vi "RoundU8.vi"(5 "Decimal places":i8, 6 "Number":u8) -> (2 "Rounded number":u8)   [LabVIEW 2017, in "GPNumeric.lvlib"]
doc: "Rounds <B>Number</B> to a number of <B>Decimal places</B>.\n\nSet <B>Decimal places</B> to a negative number to round to nearest 10, nearest 100 and so on. E.g. to round 782 to the nearest hundred, you set <B>Decimal places</B> to -2 and the <B>Rounded number</B> will be 800.\n\nThis VI is inlined.\n\n<B>Note</B> This VI uses the default IEEE 754 round-half-to-even rounding mode.\n\nSteen Schmidt\nGPower\n15/5 2014"
uses:
  GPNumeric.lvlib
  Overflow/GPOverflow.lvlib
  Overflow/Library/Mult/MultU8.vi
panel:
  # "Copyright © 2014\nGPower\nSee enclosed license file for terms and conditions"
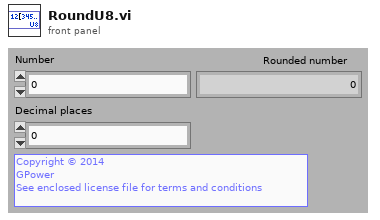
[diagram p1: front panel]
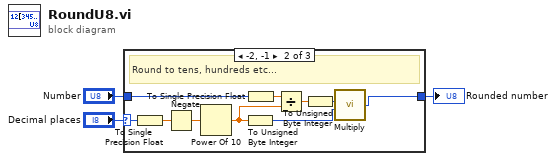
[diagram p0: block diagram]
diagram:
  n1 = case shown="-2, -1" "Decimal places" {
    selector: "Decimal places" -> [_ w8 _]
    tunnel: [_ w5 w14] -> w3
    tunnel: "Number" -> [_ w6 w14]
    frame ..-3 {
      # "Round above max value; Return zero."
    }
    frame -2, -1 {
      # "Round to tens, hundreds etc..."
      n2 = To Single Precision Float(number=w8) -> (single precision float=w7:sgl)
      n3 = Negate(x=w7) -> (-x=w13:sgl)
      n4 = Power Of 10(x=w13) -> (10^x=w4:sgl)
      n5 = To Unsigned Byte Integer(number=w4) -> (unsigned 8bit integer=w11:u8)
      n6 = To Single Precision Float(number=w6) -> (single precision float=w9:sgl)
      n7 = Divide(x=w9, y=w4) -> (x/y=w12:sgl)
      n8 = To Unsigned Byte Integer(number=w12) -> (unsigned 8bit integer=w10:u8)
      n9 = call-poly "Multiply.vi"("y"=w11, "x"=w10) -> ("x*y"=w5:u8)  [unwired: 3 in, 1 out]
    }
    frame 0.. {
      # "Round to n decimal places; return integer unchanged."
    }
  }
  "Rounded number" <- w3
